vi "JoystickSmoth.vi"(11 "joystick Value":dbl) -> (3 "new Joystick Value":dbl)   [LabVIEW 2015]
panel:
  out "input":dbl
  out "Numeric":i32
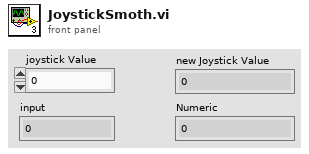
[diagram p1: front panel]
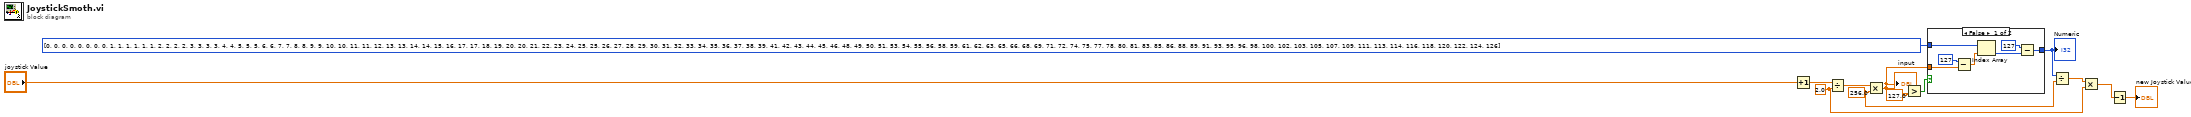
[diagram p0: block diagram]
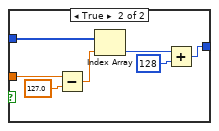
[diagram p2: hidden frame]
diagram:
  w5 = 256.0 ("y")
  w3 = 2.0 ("y")
  n1 = Increment(x="joystick Value") -> (x+1=w13:dbl)
  n2 = Divide(x=w13, y=w3) -> (x/y=w12:dbl)
  n3 = Multiply(x=w12, y=w5) -> (x*y=w8:dbl)
  "input" <- w8
  n4 = Greater?(x=w8, y=127.0) -> (0:w10:bool)
  n5 = case shown="False" w10 {
    tunnel: w8 -> [w19 w27]
    tunnel: i32[] [0, 0, 0, 0, 0, 0, 0, 0, 1, 1, 1, 1, 1, 1, 2, 2, 2, 2, 3, 3, 3, 3, 4, 4, 5, 5, 5, 6, 6, 7, 7, 8, 8, 9, 9, 10, 10, 11, 11, 12, 13, 13, 14, 14, 15, 16, 17, 17, 18, 19, 20, 20, 21, 22, 23, 24, 25, 25, 26, 27, 28, 29, 30, 31, 32, 33, 34, 35, 36, 37, 38, 39, 41, 42, 43, 44, 45, 46, 48, 49, 50, 51, 53, 54, 55, 56, 58, 59, 61, 62, 63, 65, 66, 68, 69, 71, 72, 74, 75, 77, 78, 80, 81, 83, 85, 86, 88, 89, 91, 93, 95, 96, 98, 100, 102, 103, 105, 107, 109, 111, 113, 114, 116, 118, 120, 122, 124, 126] -> [w18 w25]
    tunnel: [w14 w21] -> w6
    frame False {
      n6 = Subtract(x=127, y=w19) -> (x-y=w17:dbl)
      n7 = Index Array(array=w18, index=w17) -> (element=w15:i32)
      n8 = Subtract(x=127, y=w15) -> (x-y=w14:i32)
    }
    frame True {
      n9 = Subtract(x=w27, y=127.0) -> (x-y=w24:dbl)
      n10 = Index Array(array=w25, index=w24) -> (element=w23:i32)
      n11 = Add(x=w23, y=128) -> (x+y=w21:i32)
    }
  }
  "Numeric" <- w6
  n12 = Divide(x=w6, y=w5) -> (x/y=w4:dbl)
  n13 = Multiply(x=w4, y=w3) -> (x*y=w2:dbl)
  n14 = Decrement(x=w2) -> (x-1=→"new Joystick Value":dbl)
